vi "Set All Scripts.vi"(7 "Server Alias":string, 10 "Error In":errorcluster, 11 "All Scripts":T1[](array[typedef])) -> (2 "Error Out":errorcluster)   [LabVIEW 2013, in "TS.lvlib"]
uses:
  TS.lvlib
  LabVIEW Example/Supporting Code/Script Running.ctl
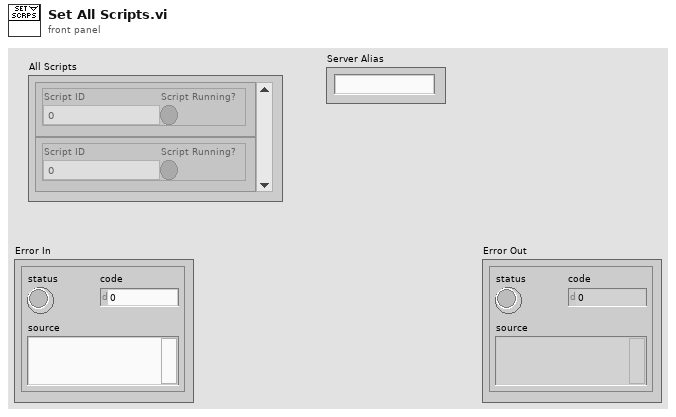
[diagram p1: front panel]
types:
  T1 = typedef "TS.lvlib/Script Running.ctl" = cluster{"Script ID":i64, "Script Running?":bool}
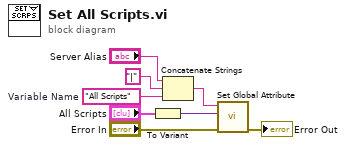
[diagram p0: block diagram]
diagram:
  w5 = "All Scripts"  # Variable Name
  n1 = To Variant(anything="All Scripts") -> (Variant=w1:variant)
  n2 = Concatenate Strings("Server Alias", "|" ("string"), w5) -> (w4:string)
  n3 = call "Set Global Attribute.vi"("Error In"="Error In", "Value"=w1, "Name"=w4) -> ("Error Out"=→"Error Out":errorcluster)  [unwired: 7 in, 1 out]
